vi "fb_lin_ctrl.vi"(0 "w":dbl, 1 "w_d":dbl, 2 "V_in":dbl, 3 "error in (no error)":errorcluster, 4 "k_p":dbl) -> (5 "u":dbl, 6 "error out":errorcluster)   [LabVIEW 2019]
panel:
  out "u_fbl":dbl
  out "e":dbl
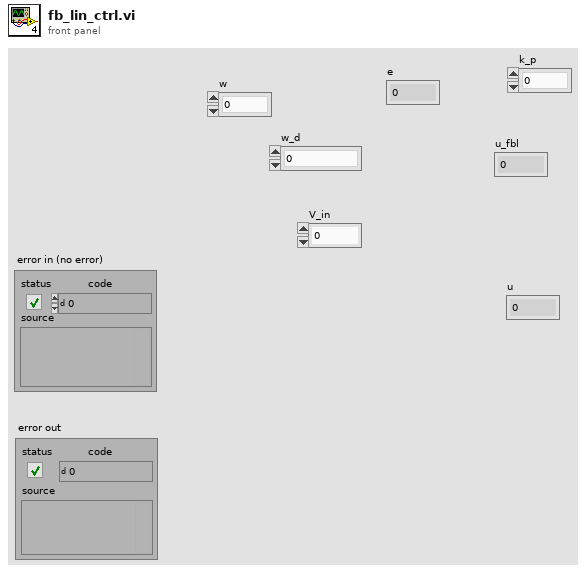
[diagram p1: front panel]
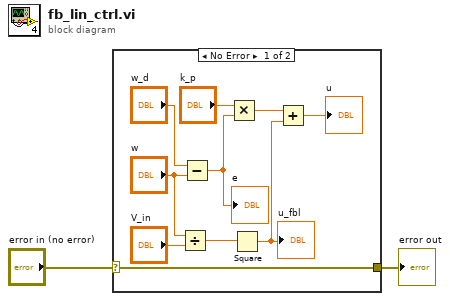
[diagram p0: block diagram]
diagram:
  n1 = case shown="No Error" "error in (no error)" {
    selector: "error in (no error)" -> [w3 w13]
    tunnel: [w3 w13] -> w1
    frame No Error {
      n2 = Divide(x="w", y="V_in") -> (x/y=w9:dbl)
      n3 = Subtract(x="w_d", y="w") -> (x-y=w5:dbl)
      "e" <- w5
      n4 = Multiply(x="k_p", y=w5) -> (x*y=w6:dbl)
      n5 = Square(x=w9) -> (x^2=w7:dbl)
      "u_fbl" <- w7
      n6 = Add(x=w6, y=w7) -> (x+y=→"u":dbl)
    }
    frame Error {
    }
  }
  "error out" <- w1
